vi "testserver.vi"() -> ()   [LabVIEW 2016]
uses:
  tls classes/connection creator/server acceptor/server acceptor.lvclass
  C:/Users/IEUser/Desktop/libasynclvtls/tls classes/connection creator/connection creator.lvclass
  tls classes/engine context/engine context.lvclass
  tls classes/connection/connection.lvclass
  tls classes/connection creator/connection creator.lvclass
panel:
  out "output cluster":cluster{"error code":i32, "data":string}
  out "error out":errorcluster
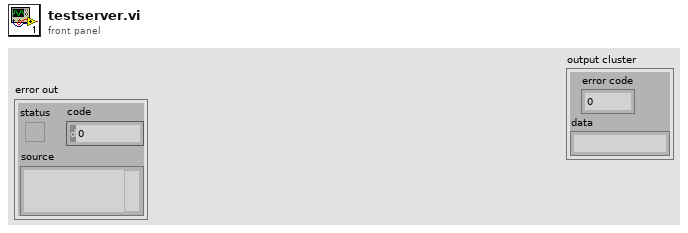
[diagram p1: front panel]
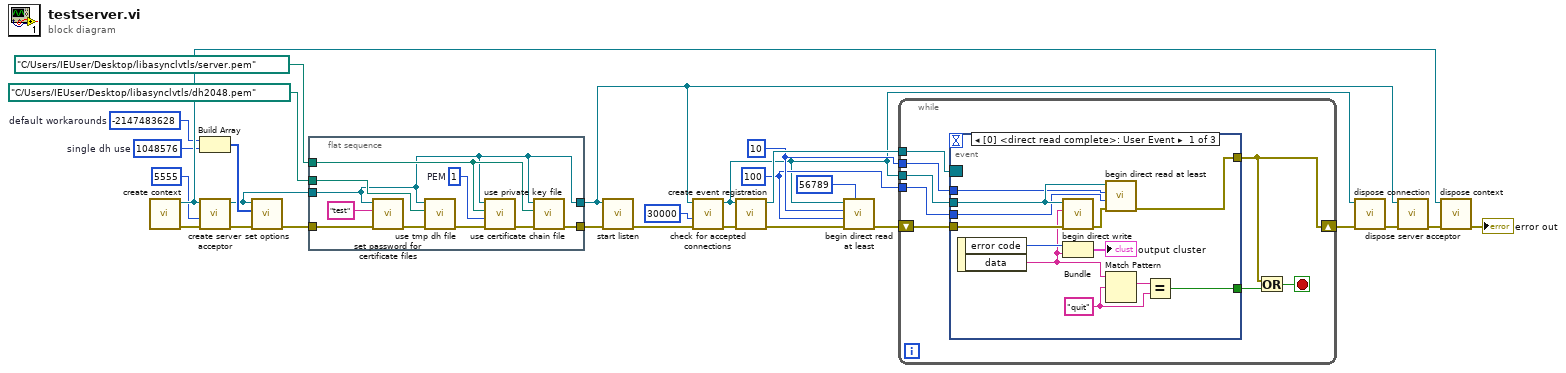
[diagram p0: block diagram]
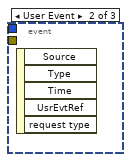
[diagram p2: hidden frame]
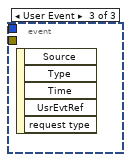
[diagram p3: hidden frame]
diagram:
  w15 = -2147483628  # default workarounds
  w16 = 1048576  # single dh use
  w6 = 100 ("bytes to read")
  w7 = 10 ("bytes to read")
  n1 = call "create context.vi"() -> ("error out"=w19:errorcluster, "engine context out"=w18:refnum<class "engine context.lvclass">)  [unwired: 10 in]
  n2 = Build Array(w15, w16) -> (w3:i32[])
  n3 = call "create server acceptor.vi"("error in"=w19, "port"=u16 5555, "engine context in"=w18) -> ("error out"=w17:errorcluster, "server acceptor out"=w2:refnum<class "server acceptor.lvclass">)  [unwired: 7 in]
  n4 = call "set options.vi"("error in"=w17, "options"=w3, "connection creator in"=w2) -> ("error out"=w14:errorcluster)  [unwired: 8 in]
  n5 = flat-sequence {
    tunnel: w14 -> [w37]
    tunnel: path "C:/Users/IEUser/Desktop/libasynclvtls/dh2048.pem" ("tmp dh file") -> [w35]
    tunnel: path "C:/Users/IEUser/Desktop/libasynclvtls/server.pem" ("cert chain file") -> [w34]
    tunnel: [w32] -> w11
    tunnel: w2 -> [w31]
    tunnel: [w31] -> w1
    frame #0 {
      w33 = 1  # PEM
      n6 = call "set password for certificate files.vi"("error in"=w37, "password"="test" ("file"), "connection creator in"=w31) -> ("error out"=w30:errorcluster)  [unwired: 8 in]
      n7 = call "use tmp dh file.vi"("error in"=w30, "tmp dh file"=w35, "connection creator in"=w31) -> ("error out"=w29:errorcluster)  [unwired: 8 in]
      n8 = call "use private key file.vi"("error in"=w29, "format"=w33, "private key file"=w34, "connection creator in"=w31) -> ("error out"=w28:errorcluster)  [unwired: 7 in]
      n9 = call "use certificate chain file.vi"("error in"=w28, "cert chain file"=w34, "connection creator in"=w31) -> ("error out"=w32:errorcluster)  [unwired: 8 in]
    }
  }
  n10 = call "start listen.vi"("error in"=w11, "server acceptor in"=w1) -> ("error out"=w10:errorcluster)  [unwired: 9 in]
  n11 = call "check for accepted connections.vi"("error in"=w10, "timeout"=30000, "server acceptor in"=w1) -> ("error out"=w9:errorcluster, "connection"=w5:refnum<class "connection.lvclass">)  [unwired: 7 in]
  n12 = call "create event registration.vi"("error in"=w9, "connection in"=w5) -> ("error out"=w26:errorcluster, "Event Registration Refnum"=w27:refnum<event-registration>)  [unwired: 8 in]
  n13 = call "begin direct read at least.vi"("id"=u32 56789, "error in"=w26, "max bytes to read"=w6, "min bytes to read"=w7, "connection in"=w5) -> ("error out"=w24:errorcluster)  [unwired: 6 in]
  n14 = while {
    tunnel: w27 -> [w45]
    shift-right: [w39] -> w21
    shift-left: w24 -> [w44]
    tunnel: w5 -> [w43]
    tunnel: w7 -> [w42]
    tunnel: w6 -> [w41]
    stop <- w40 stop-if-true
    n15 = event shown="[0] <direct read complete>: User Event" {
      selector: w45 -> [_ _ _]
      dyn-events: _ -> [_ _ _]
      timeout: _ -> [_ _ _]
      tunnel: w44 -> [w55 _ _]
      tunnel: w43 -> [w52 _ _]
      tunnel: [w53 _ _] -> w39
      tunnel: w42 -> [w51 _ _]
      tunnel: w41 -> [w50 _ _]
      tunnel: [w49 _ _] -> w38
      event User Event {
        w46 = "quit" ("y")
        n16 = event-data() -> ("error code"=w57:i32, "data"=w48:string)  [unwired: 1 in]
        n17 = call "begin direct write.vi"("error in"=w55, "data"=w48, "connection in"=w52) -> ("error out"=w54:errorcluster)  [unwired: 8 in]
        n18 = Bundle("error code"=w57, "data"=w48) -> (→"output cluster":cluster{"error code":i32, "data":string})  [unwired: 1 in]
        n19 = call "begin direct read at least.vi"("error in"=w54, "max bytes to read"=w50, "min bytes to read"=w51, "connection in"=w52) -> ("error out"=w53:errorcluster)  [unwired: 7 in]
        n20 = Match Pattern(string=w48, regular expression=w46) -> (match substring=w47:string)  [unwired: 1 in, 3 out]
        n21 = Equal?(x=w47, y=w46) -> (x = y?=w49:bool)
      }
      event User Event {
        n22 = event-data() -> ()  [unwired: 1 in, 5 out]
      }
      event User Event {
        n23 = event-data() -> ()  [unwired: 1 in, 5 out]
      }
    }
    n24 = Or(x=w39, y=w38) -> (x .or. y?=w40:bool)
  }
  n25 = call "dispose connection.vi"("error in"=w21, "connection in"=w5) -> ("error out"=w23:errorcluster)  [unwired: 9 in]
  n26 = call "dispose server acceptor.vi"("error in"=w23, "server acceptor in"=w1) -> ("error out"=w22:errorcluster)  [unwired: 9 in]
  n27 = call "dispose context.vi"("error in"=w22, "engine context out"=w18) -> ("error out"=→"error out":errorcluster)  [unwired: 9 in]
